vi "motion_control_parameter.vi"() -> ()   [LabVIEW 2018]
panel:
  in  "Kp":dbl
  in  "shutoff":dbl
  in  "运动模拟信号增益":dbl
  in  "unlock":dbl[](array[numeric])
  in  "error":dbl
  in  "shengguang":dbl
  in  "atti_standby_position":dbl
  in  "atti_reset_position":dbl
  in  "LVDT信号":dbl[](array[numeric])
  in  "ScopeData_Unpack":dbl[][](array[numeric])
  in  "数据存储？":bool
  out "ScopeFinish":bool
  in  "Time":dbl[](array[numeric])
  in  "ScopeData":dbl[][](array[numeric])
  out "Encoded_Signal_Data":dbl[](array[numeric])
  in  "ShowClock":dbl
  out "Show_Select_Signal":i32[](array[numeric])
  in  "Api_Port":i32
  in  "单缸错误限制":dbl[](array[numeric])
  in  "位置反馈下限":dbl[](array[numeric])
  in  "位置反馈上限":dbl[](array[numeric])
  in  "方波通道选择":bool[](array[boolean])
  in  "随机波通道选择":bool[](array[boolean])
  in  "任意波滤波通道选择":dbl
  in  "随机波幅值":dbl[](array[numeric])
  in  "方波信号偏移":dbl[](array[numeric])
  in  "方波信号周期":dbl[](array[numeric])
  in  "方波信号幅值":dbl[](array[numeric])
  out "正弦信号通道选择":bool[](array[boolean])
  in  "位移传感器原始参数":dbl[](array[numeric])
  out "ErrorCodeMotion":bool[](array[boolean])
  in  "表示码":dbl
  in  "receive_data":dbl[](array[numeric])
  in  "System_oil_pressure":dbl
  in  "System_oil_tempeture":dbl
  in  "Sine_bias":dbl[](array[numeric])
  in  "Attri_from_host2":dbl[](array[numeric])
  in  "Sine_freq":dbl[](array[numeric])
  in  "Sine_phase":dbl[](array[numeric])
  in  "Sine_amp":dbl[](array[numeric])
  in  "Heartbeat":dbl
  in  "Reset":dbl
  in  "recheck":dbl
  in  "actu_atti":dbl
  in  "Ready":dbl
  in  "continue_motion":bool
  out "di_coming":bool[](array[boolean])
  in  "alarm":bool
  in  "Switch":dbl
  in  "Startcmd":dbl
  in  "SignalSelect":dbl
  # "方波信号"
  # "常值信号"
  # "正弦信号参数"
  # "频率"
  # "幅值"
  # "相位"
  # "偏移"
  # "随机波"
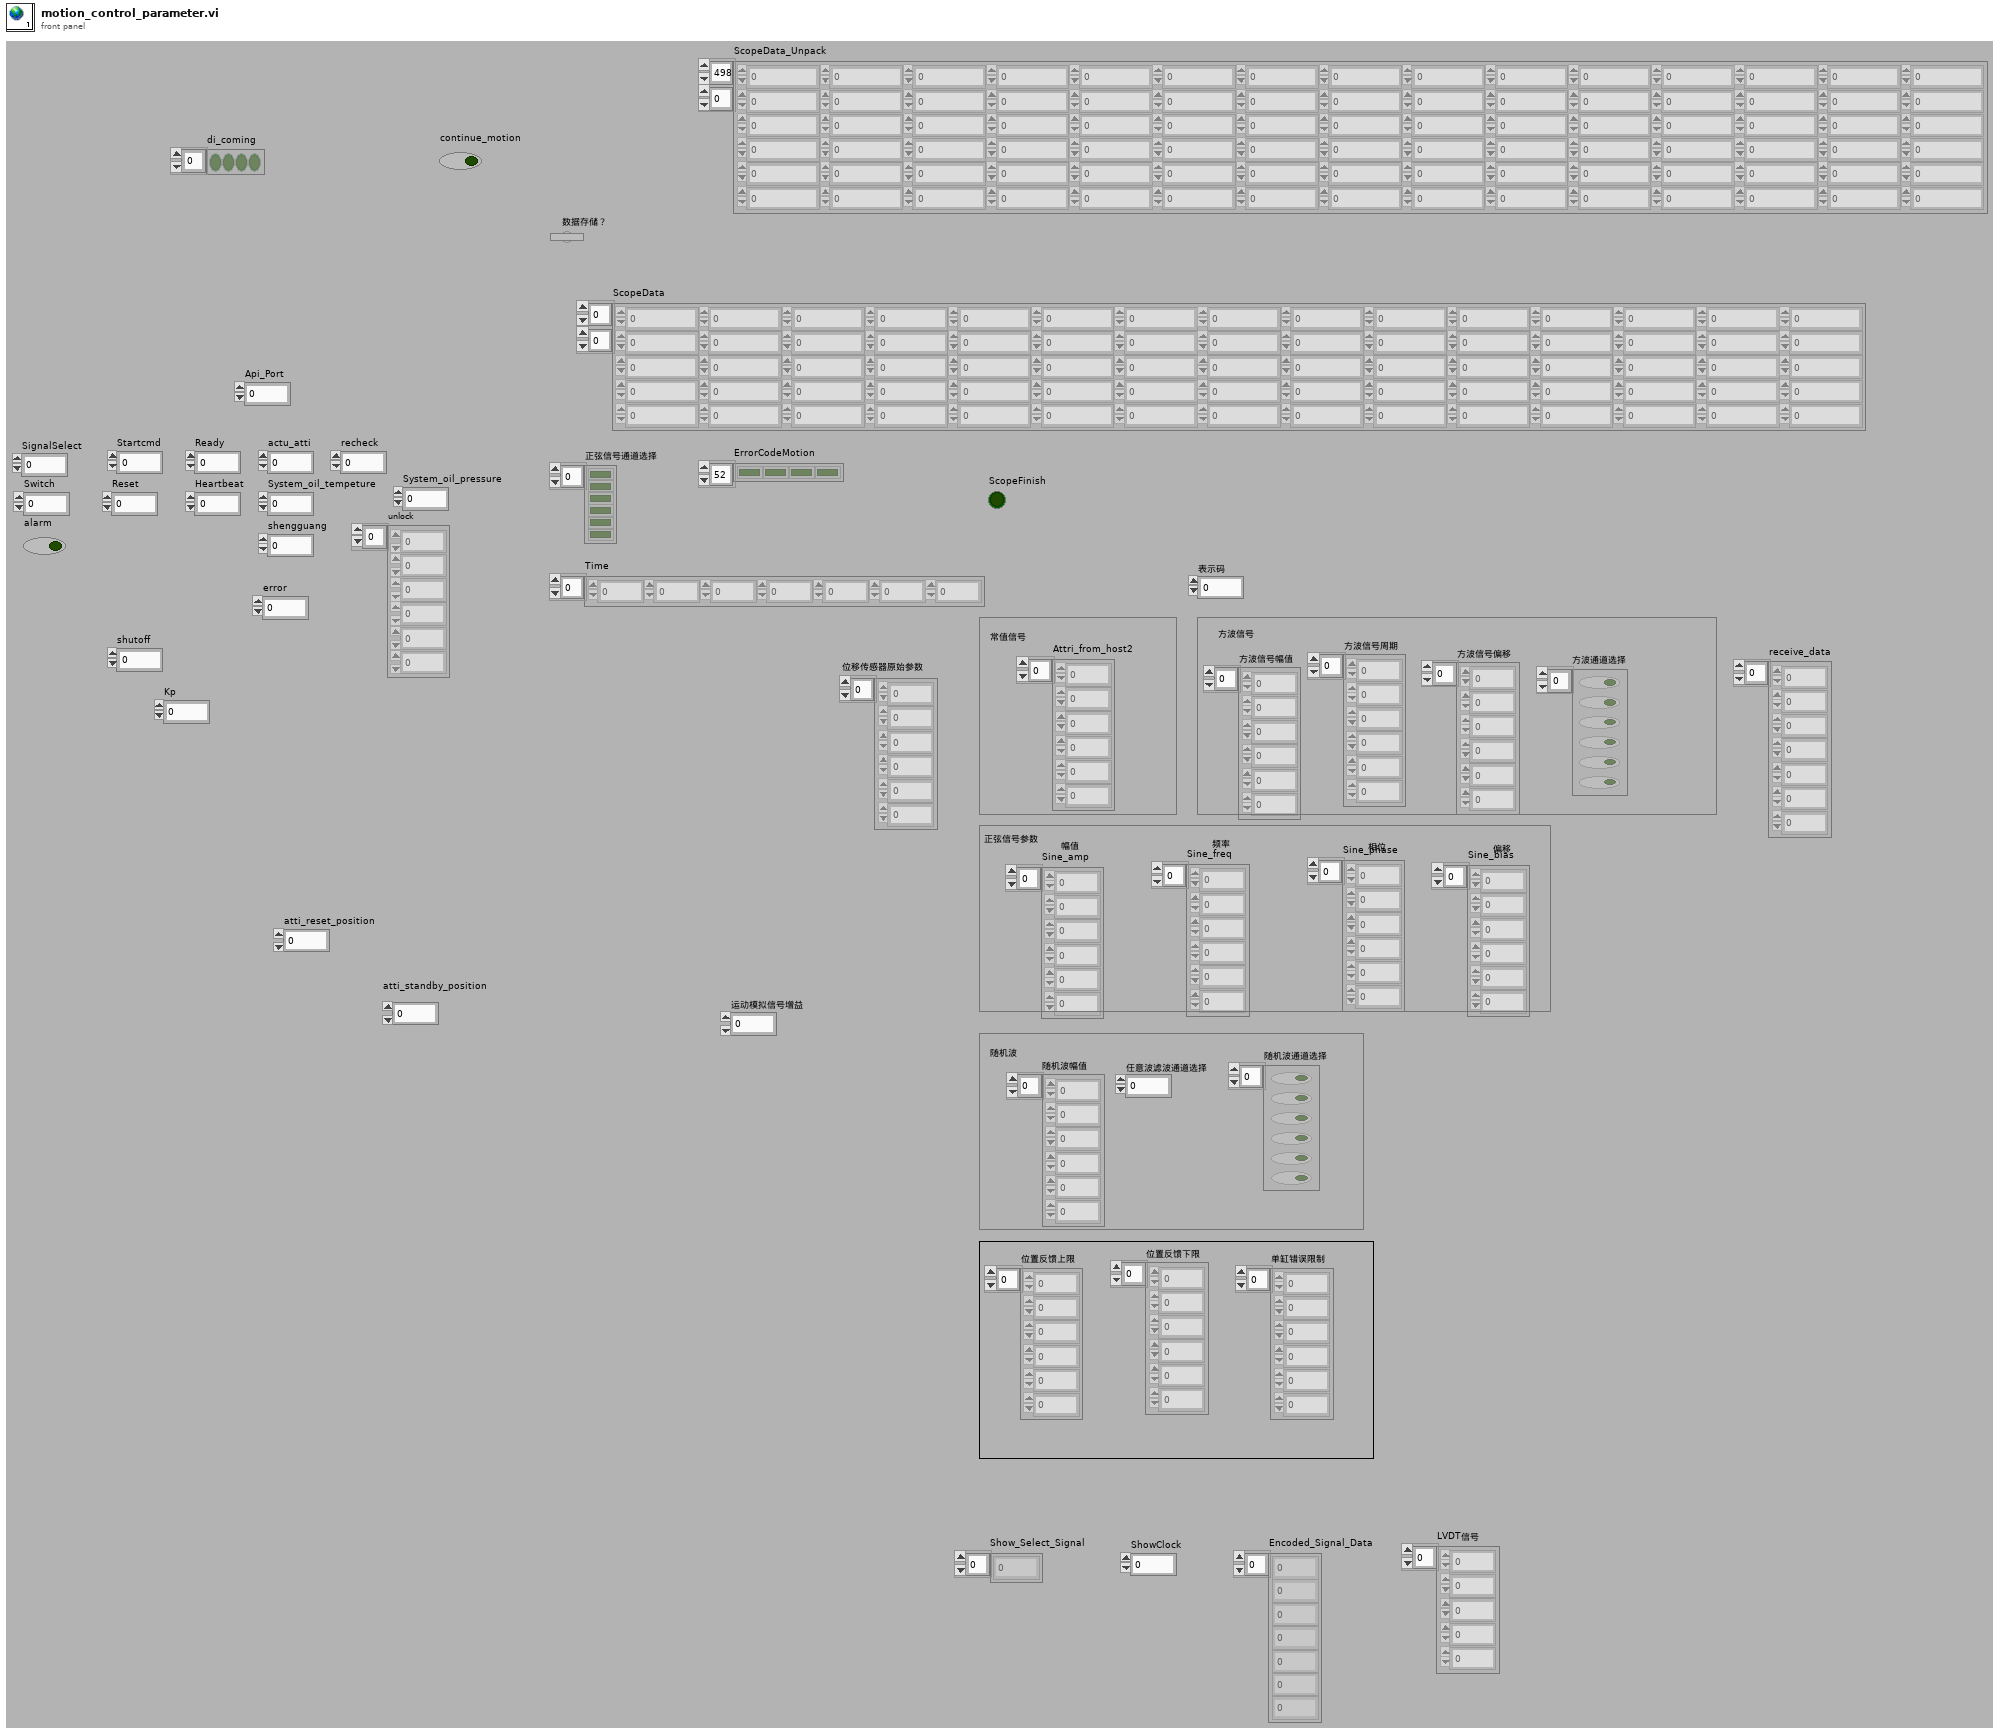
[diagram p1: front panel]
diagram:
